vi "Read Batch Profile Storage Data.vi"(0 "Device ID (0)":i32, 5 "Read Req":T6, 7 "Data Size (0: Auto Size)":u32, 11 "error in (no error)":errorcluster) -> (2 "Storage Time Cnt":u32, 3 "Profile Info":T7, 4 "Device ID out":i32, 6 "Storage Data":u32[](array[numeric]), 8 "Storage Rsp":T4, 10 "Measure Data":T1[](array[typedef]) {"Judge Result" items=["HI", "GO", "LO", "ALARM"]; "Data Info" items=["VALID", "ALARM", "WAIT"]}, 14 "Storage Info":T8, 15 "error out":errorcluster)   [LabVIEW 8.6, in "Keyence LJ-V7000.lvlib"]
doc: "When the storage target setting is profile, this function gets the stored profile data. (Batch setting: on)\n\nIf the data specified by \"<B>Read Batch Top Profile No</B>\" in <B>Read Req</B> has not been accumulated, one item of the newest data that has been accumulated is returned.\n\n<B>Note</B>:\nFor the details on the data stored in the profile data (storage order and size), refer to <B>10.3</B> in a manual of measuring instrument drivers.\n\nIf Compression(timse axis) is ON, use <B>Read Profile Storage Data</B> VI."
uses:
  Keyence LJ-V7000.lvlib
  constant/Driver VI No.ctl
  Clusters/Storage Info.ctl
  Clusters/Time.ctl
  Clusters/Profile Info.ctl
  Clusters/Read Batch Profile Storage Rsp.ctl
  Private/vi/Low Level/Make DLL Param(Read Batch Profile Storage Rsp).vi
  Private/vi/Low Level/Make VI Param(Read Batch Profile Storage Rsp).vi
  constant/Judge Result.ctl
  constant/Measure Data Info.ctl
  Clusters/Measure Data.ctl
  Clusters/Read Batch Profile Storage Req.ctl
panel:
  # "(c) 2012 KEYENCE CORPORATION.  ALL RIGHTS RESERVED."
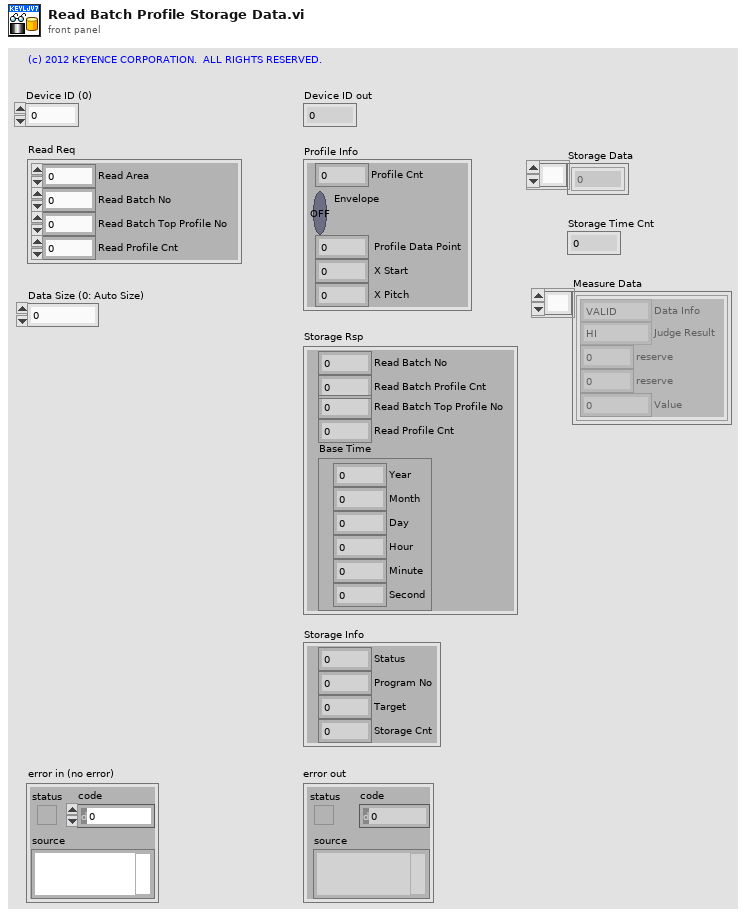
[diagram p1: front panel]
types:
  T1 = typedef "Keyence LJ-V7000.lvlib/Measure Data.ctl" = cluster{"Data Info":T2, "Judge Result":T3, "reserve":u8, "reserve":u8, "Value":sgl}
  T2 = typedef "Keyence LJ-V7000.lvlib/Measure Data Info.ctl" = u8
  T3 = typedef "Keyence LJ-V7000.lvlib/Judge Result.ctl" = u8
  T4 = typedef "Keyence LJ-V7000.lvlib/Read Batch Profile Storage Rsp.ctl" = cluster{"Read Batch No":u32, "Read Batch Profile Cnt":u32, "Read Batch Top Profile No":u32, "Read Profile Cnt":u8, "Base Time":T5}
  T5 = typedef "Keyence LJ-V7000.lvlib/Time.ctl" = cluster{"Year":u8, "Month":u8, "Day":u8, "Hour":u8, "Minute":u8, "Second":u8}
  T6 = typedef "Keyence LJ-V7000.lvlib/Read Batch Profile Storage Req.ctl" = cluster{"Read Area":u32, "Read Batch No":u32, "Read Batch Top Profile No":u32, "Read Profile Cnt":u8}
  T7 = typedef "Keyence LJ-V7000.lvlib/Profile Info.ctl" = cluster{"Profile Cnt":u8, "Envelope":bool, " Profile Data Point":u16, " X Start":i32, " X Pitch":i32}
  T8 = typedef "Keyence LJ-V7000.lvlib/Storage Info.ctl" = cluster{"Status":u8, "Program No":u8, "Target":u8, "Storage Cnt":u32}
  T9 = typedef "Keyence LJ-V7000.lvlib/Driver VI No.ctl" = enum16{"Initialize", "Close", "Reboot Controller", "Return to Factory State", "Get System Error", "Clear System Error", "Trigger", "Start Batch Measurements", "Stop Batch Measurements", "Auto Zero", "Timing", "Reset", "Clear Memory", "Set Setting", "Get Setting", "Initialize Setting", "Reflect Setting", "Update Write Settings Area", "Check Status of Saving to Save Area", "Set Time", "Get Time", "Change Program", "Read Active Program Number", "Read Measurement Data", "Read Profiles(for High-Speed Mode)", "Read Batch Profiles(for High-Speed Mode)", "Read Profiles(for Advanced Mode)", "Read Batch Profiles(for Advanced Mode)", "Start Storage", "Stop Storage", "Read Storage Status", "Read Data Storage Data", "Read Profile Storage Data", "Read Batch Profile Storage Data", "Start High-Speed Data Communication", "Stop High-Speed Data Communication", "Read Profiles(for High-Speed Communication)"}
  T10 = cluster{"reserved":u8, "reserved":u8, "reserved":u8, "reserved":u8, "Read Area":u32, "Read Batch No":u32, "Read Batch Top Profile No":u32, "Read Profile Cnt":u8, "reserved":u8, "reserved":u8, "reserved":u8}
  T11 = cluster{"Status":u8, "Program No":u8, "Target":u8, "reserved":u8, "reserved":u8, "reserved":u8, "reserved":u8, "reserved":u8, "Storage Cnt":u32}
  T12 = cluster{"Read Batch No":u32, "Read Batch Profile Cnt":u32, "Read Batch Top Profile No":u32, "Read Profile Cnt":u8, "reserved":u8, "reserved":u8, "reserved":u8, "pTime":cluster{"Year":u8, "Month":u8, "Day":u8, "Hour":u8, "Minute":u8, "Second":u8, "reserved":u8, "reserved":u8}}
  T13 = cluster{"Profile Cnt":u8, u8, "reserve":u8, "reserve":u8, " Profile Data Point":u16, "reserve":u8, "reserve":u8, " X Start":i32, " XPitch":i32}
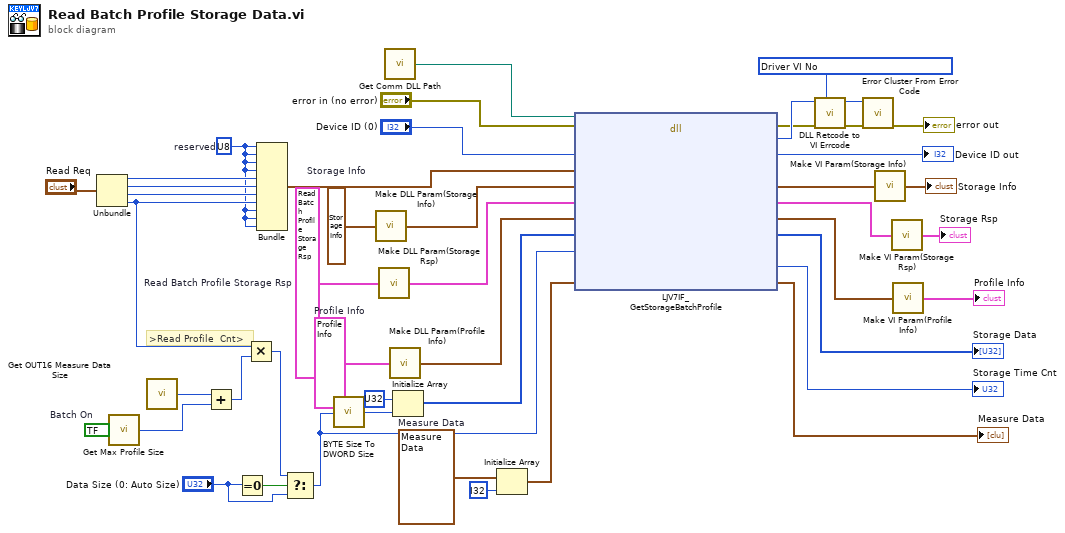
[diagram p0: block diagram]
diagram:
  w16 = T1 ?  # Measure Data
  w21 = T4 ?  # Read Batch Profile Storage Rsp
  w26 = bool ?  # Batch On
  w31 = T7 ?  # Profile Info
  w38 = T8 ?  # Storage Info
  w22 = u8 ?  # reserved
  # ">Read Profile  Cnt>"
  n1 = Unbundle("Read Req") -> ("Read Area"=w41:u32, "Read Batch No"=w40:u32, "Read Batch Top Profile No"=w32:u32, "Read Profile Cnt"=w23:u8)
  n2 = call "Get Max Profile Size.vi"("Batch On-Off"=w26) -> ("Profile Size"=w10:u32)  [unwired: 4 in]
  n3 = call "Get OUT16 Measure Data Size.vi"() -> ("OUT16 Measure Data Size"=w18:u32)  [unwired: 1 in]
  n4 = Add(x=w18, y=w10) -> (x+y=w17:u32)
  n5 = Equal To 0?(x="Data Size (0: Auto Size)") -> (x = 0?=w27:bool)
  n6 = Multiply(x=w23, y=w17) -> (x*y=w9:u32)
  n7 = Bundle("reserved"=w22, "reserved"=w22, "reserved"=w22, "reserved"=w22, "Read Area"=w41, "Read Batch No"=w40, "Read Batch Top Profile No"=w32, "Read Profile Cnt"=w23, "reserved"=w22, "reserved"=w22, "reserved"=w22) -> (w39:T10)  [unwired: 1 in]
  n8 = Select(t=w9, s=w27, f="Data Size (0: Auto Size)") -> (s? t:f=w7:u32)
  n9 = call "BYTE Size To DWORD Size.vi"("BYTE Size"=w7) -> ("DWORD Size"=w11:u32)
  n10 = call "Make DLL Param(Storage Info).vi"("Storage Info"=w38) -> ("pStorageInfo"=w37:T11)
  n11 = call-poly "Make DLL Param(Storage Rsp).vi"("Read Batch Profile Storage Rsp"=w21) -> ("pRsp"=w34:T12)
  n12 = call "Get Comm DLL Path.vi"() -> ("Comm DLL Path"=w44:path)  [unwired: 1 in]
  n13 = call "Make DLL Param(Profile Info).vi"("Profile Info"=w31) -> ("DLL Parameter"=w30:T13)
  n14 = Initialize Array(u32 ?, w11) -> (w8:u32[])
  n15 = Initialize Array(w16, i32 ? ("次元サイズ")) -> (w14:T1[])
  n16 = dll-call lib="C:/Program Files/National Instruments/LabVIEW 2011/instr.lib/Keyence LJ-V7000/LJV7_IF.*" fn="LJV7IF_GetStorageBatchProfile"(path in=w44, error in="error in (no error)", "lDeviceId"="Device ID (0)", "pReq"=w39, "pStorageInfo"=w37, "pRsp"=w34, "pProfileInfo"=w30, "pdwData"=w8, "dwDataSize"=w7, "pMeasureData"=w14) -> (error out=w3:errorcluster, "lRetCode"=w4:i32, "lDeviceId"=→"Device ID out":i32, "pStorageInfo"=w35:T11, "pRsp"=w33:T12, "pProfileInfo"=w28:T13, "pdwData"=→"Storage Data":u32[], "pdwTimeOffset"=→"Storage Time Cnt":u32, "pMeasureData"=→"Measure Data":T1[])  [unwired: 4 in, 1 out]
  n17 = call "DLL Retcode to VI Errcode.vi"("Driver VI No"=T9 ?, "error in (no error)"=w3, "DLL Return Code"=w4) -> ("error out"=w6:errorcluster, "VI Error Code"=w5:i32)  [unwired: 7 in]
  n18 = call <vilib>:"Error Cluster From Error Code.vi"("error in (no error)"=w6, "error code (0)"=w5) -> ("error out"=→"error out":errorcluster)  [unwired: 7 in]
  n19 = call "Make VI Param(Storage Info).vi"("pStorageInfo"=w35) -> ("Storage Info"=→"Storage Info":T8)
  n20 = call-poly "Make VI Param(Storage Rsp).vi"("pRsp"=w33) -> ("Read Batch Profile Storage Rsp"=→"Storage Rsp":T4)
  n21 = call "Make VI Param(Profile Info).vi"("pProfileInfo"=w28) -> ("Profile Info"=→"Profile Info":T7)
